vi "EXAMPLE.vi"(8 "error in (no error)":errorcluster, 11 "PSP-405 resource in":refnum<visa-resource-name>) -> (0 "error out":errorcluster)   [LabVIEW 2017, in "GW Instek PSP-405.lvlib"]
uses:
  GW Instek PSP-405.lvlib
panel:
  out "voltage value out":dbl
  in  "voltage value in":dbl
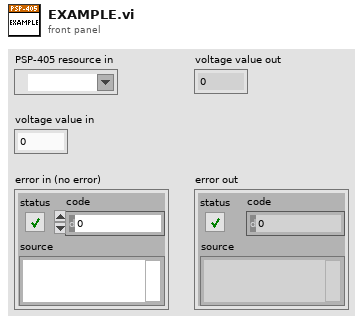
[diagram p1: front panel]
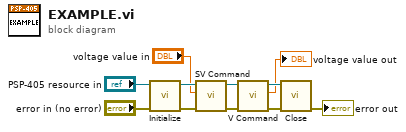
[diagram p0: block diagram]
diagram:
  n1 = call "Initialize.vi"("error in (no error)"="error in (no error)", "PSP-405 resource in"="PSP-405 resource in") -> ("error out"=w7:errorcluster, "PSP-405 resource out"=w8:refnum<visa-resource-name>)  [unwired: 8 in]
  n2 = call "SV Command.vi"("error in (no error)"=w7, "voltage value"="voltage value in", "PSP-405 resource in"=w8) -> ("error out"=w6:errorcluster, "PSP-405 resource out"=w3:refnum<visa-resource-name>)  [unwired: 7 in]
  n3 = call "V Command.vi"("error in (no error)"=w6, "PSP-405 resource in"=w3) -> ("error out"=w4:errorcluster, "voltage value"=→"voltage value out":dbl, "PSP-405 resource out"=w2:refnum<visa-resource-name>)  [unwired: 6 in, 1 out]
  n4 = call "Close.vi"("error in (no error)"=w4, "PSP-405 resource in"=w2) -> ("error out"=→"error out":errorcluster)  [unwired: 9 in]
